vi "Get Cursors.vi"(9 "tag info not from game manual":dbl[][](array[numeric]), 10 "tags":T1(array[cluster]), 11 "Cluster":T3) -> (3 "Array":T2(array[cluster]))   [LabVIEW 2025]
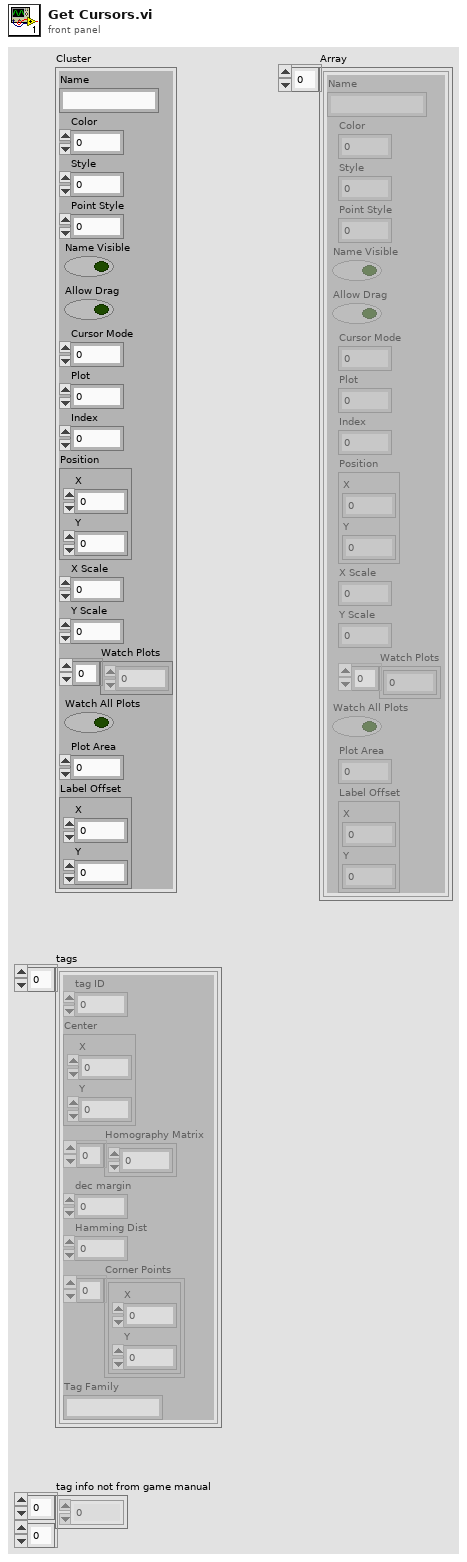
[diagram p1: front panel]
types:
  T1 = cluster{"tag ID":i32, "Center":cluster{"X":dbl, "Y":dbl}, "Homography Matrix":dbl[], "dec margin":dbl, "Hamming Dist":i32, "Corner Points":cluster{"X":dbl, "Y":dbl}[], "Tag Family":string}[]
  T2 = cluster{"Name":string, "Color":u32, "Style":i32, "Point Style":i32, "Name Visible":bool, "Allow Drag":bool, "Cursor Mode":u32, "Plot":i32, "Index":i32, "Position":cluster{"X":dbl, "Y":dbl}, "X Scale":u32, "Y Scale":u32, "Watch Plots":i32[], "Watch All Plots":bool, "Plot Area":i32, "Label Offset":cluster{"X":i32, "Y":i32}}[]
  T3 = cluster{"Name":string, "Color":u32, "Style":i32, "Point Style":i32, "Name Visible":bool, "Allow Drag":bool, "Cursor Mode":u32, "Plot":i32, "Index":i32, "Position":cluster{"X":dbl, "Y":dbl}, "X Scale":u32, "Y Scale":u32, "Watch Plots":i32[], "Watch All Plots":bool, "Plot Area":i32, "Label Offset":cluster{"X":i32, "Y":i32}}
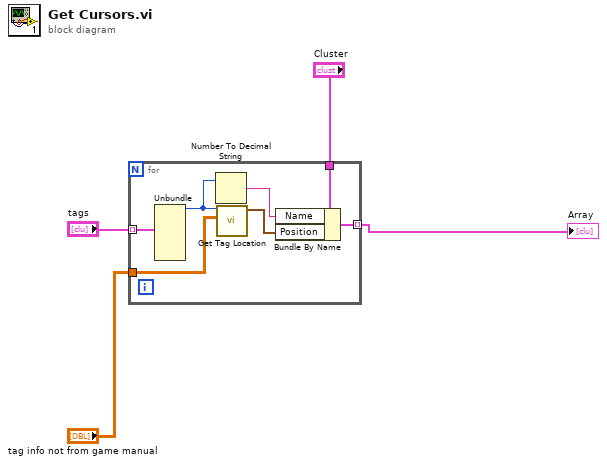
[diagram p0: block diagram]
diagram:
  n1 = for {
    tunnel: "tags" -> [w11] mode=indexing
    tunnel: "tag info not from game manual" -> [w10]
    tunnel: "Cluster" -> [w9]
    tunnel: [w7] -> w3 mode=indexing
    n2 = Unbundle(w11) -> ("tag ID"=w5:i32)  [unwired: 6 out]
    n3 = Number To Decimal String(number=w5) -> (decimal integer string=w6:string)  [unwired: 1 in]
    n4 = call "Get Tag Location.vi"("tag info"=w10, "tag ID"=w5) -> ("field locations (ft)"=w8:cluster{"X":dbl, "Y":dbl})  [unwired: 8 in, 1 out]
    n5 = Bundle By Name(cluster=w9, "Name"=w6, "Position"=w8) -> (w7:T3)
  }
  "Array" <- w3
